vi "VFH-View-libreVNA.vi"() -> ()   [LabVIEW 2020, in "VFH-VNA_File_Handler.lvlib"]
uses:
  VFH-VNA_File_Handler.lvlib
panel:
  out "Waveform Graph":dbl[][](graph)
  out "Raw 2":T1(graph)
  in  "libre":path=path "C:/projects/UNI/VNA/MiniVNA/20240625-162312-Vann/Vann.txt"
  out "Raw":T1(graph)
  in  "water":path=path "C:/projects/UNI/VNA/MiniVNA/20240625-162312-Vann/Vann.txt"
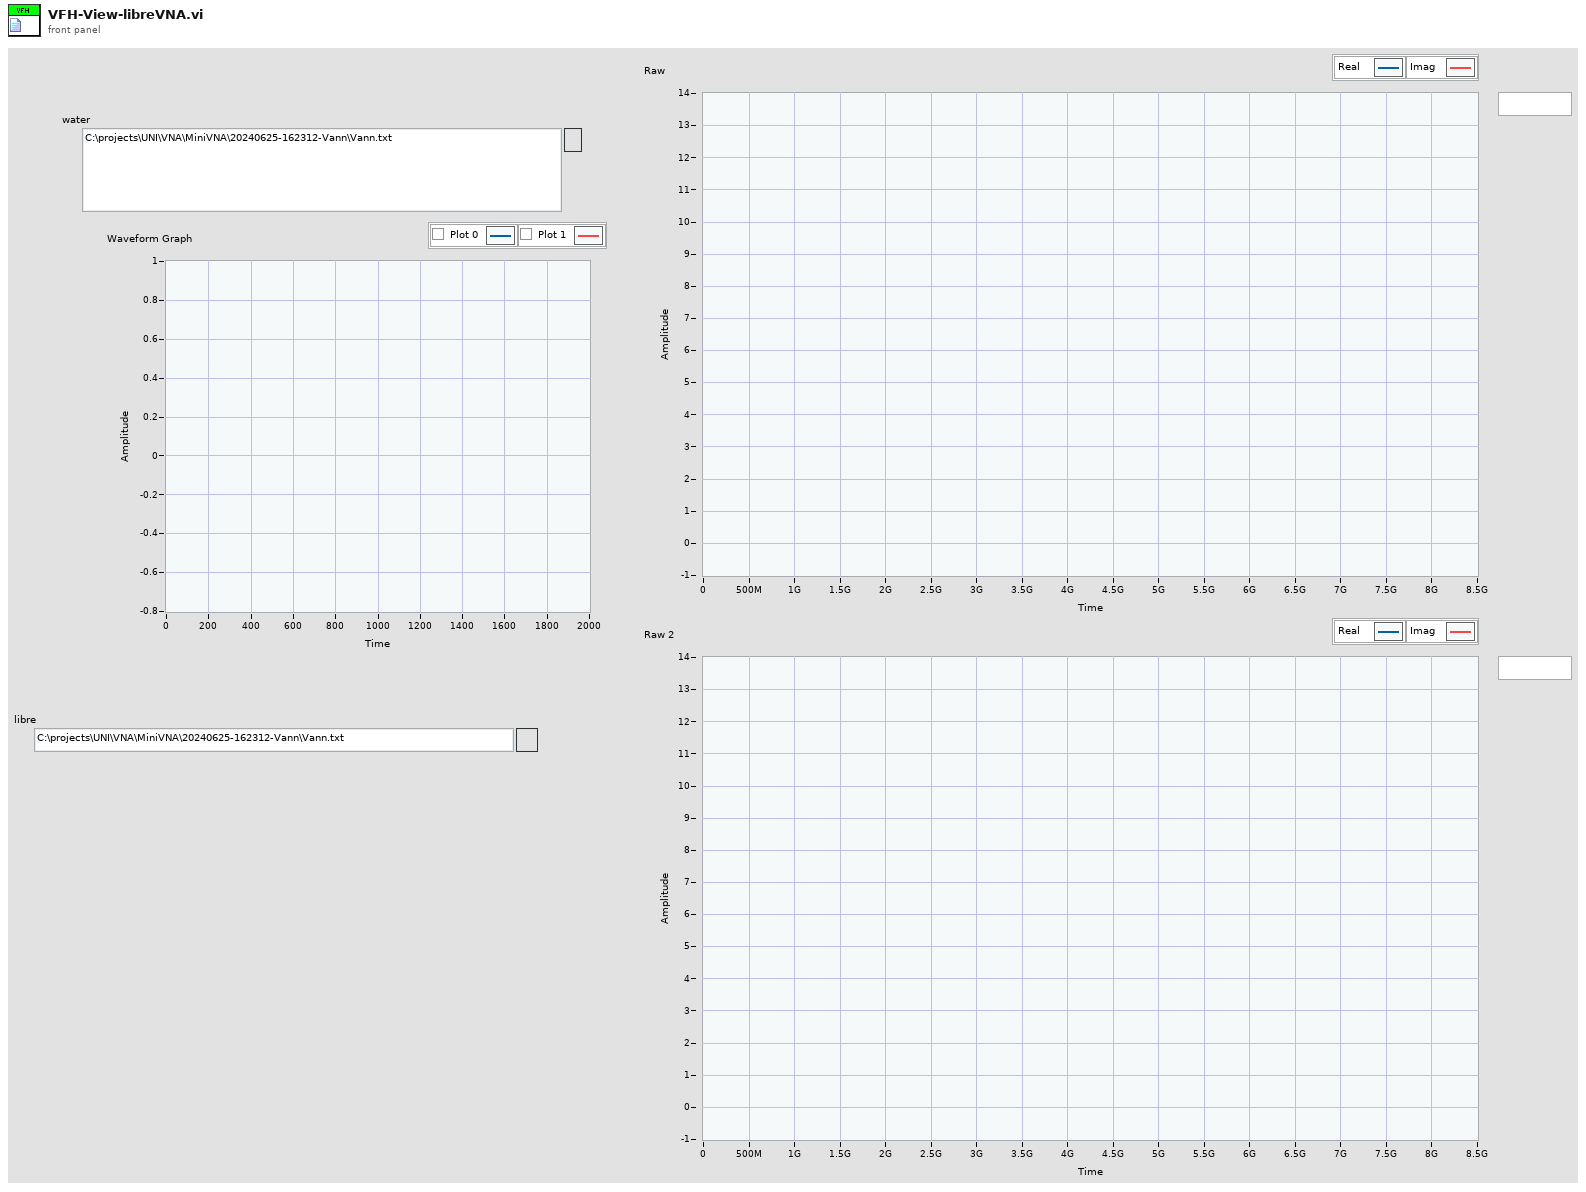
[diagram p1: front panel]
types:
  T1 = cluster{"Frequency":dbl[], "Reflection R":dbl[]}[]
  T2 = typedef "VFH-VNA_File_Handler.lvlib/VFH-file_cluster-NanoVNA.ctl" = cluster{"Frequency":dbl[], "S11_Real":dbl[], "S11_Imag":dbl[], "S21_Real":dbl[], "S21_Imag":dbl[], "S12_Real":dbl[], "S12_Imag":dbl[], "S22_Real":dbl[], "S22_Imag":dbl[]}
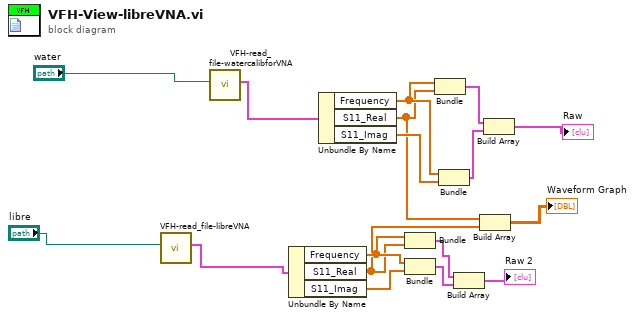
[diagram p0: block diagram]
diagram:
  n1 = call "VFH-read_file-libreVNA.vi"("file path (dialog if empty)"="libre") -> ("output cluster"=w9:T2)  [unwired: 9 in, 1 out]
  n2 = call "VFH-read_file-watercalibforVNA.vi"("file path (dialog if empty)"="water") -> ("output cluster"=w5:T2)  [unwired: 9 in, 1 out]
  n3 = Unbundle By Name(w9) -> ("Frequency"=w8:dbl[], "S11_Real"=w2:dbl[], "S11_Imag"=w10:dbl[])
  n4 = Unbundle By Name(w5) -> ("Frequency"=w4:dbl[], "S11_Real"=w3:dbl[], "S11_Imag"=w17:dbl[])
  n5 = Bundle("Frequency"=w8, "S11_Real"=w2) -> (w7:cluster{"Frequency":dbl[], "S11_Real":dbl[]})  [unwired: 1 in]
  n6 = Bundle("Frequency"=w8, "S11_Imag"=w10) -> (w11:cluster{"Frequency":dbl[], "S11_Imag":dbl[]})  [unwired: 1 in]
  n7 = Bundle("Frequency"=w4, "S11_Real"=w3) -> (w16:cluster{"Frequency":dbl[], "S11_Real":dbl[]})  [unwired: 1 in]
  n8 = Bundle("Frequency"=w4, "S11_Imag"=w17) -> (w15:cluster{"Frequency":dbl[], "S11_Imag":dbl[]})  [unwired: 1 in]
  n9 = Build Array(w7, w11) -> (→"Raw 2":cluster{"Frequency":dbl[], "S11_Imag":dbl[]}[])
  n10 = Build Array(w3, w2) -> (→"Waveform Graph":dbl[][])
  n11 = Build Array(w16, w15) -> (→"Raw":cluster{"Frequency":dbl[], "S11_Imag":dbl[]}[])
